vi "Scanning Setting.vi"() -> ()   [LabVIEW 2012]
panel:
  in  "Peizo Amp":dbl
  in  "Peizo Offset":dbl=6.0
  in  "Z Slice number":dbl=10.0
  in  "Single Line Scan":bool
  in  "Z freq":dbl=100.0
  in  "S freq":dbl=1000.0
  in  "S-Angle Correction Z":dbl=-0.41789996905297544
  in  "S-Angle Correction S":dbl=1.4178999690529754
  in  "Z-Offset":dbl=-1.0299401197604787
  in  "S-Offset":dbl=-2.175438596491228
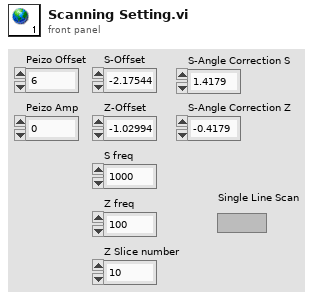
[diagram p1: front panel]
diagram:
